vi "InitControls.vi"(8 "error in (no error)":errorcluster, 9 "TestCloneAPI Reference":refnum<vi>, 11 "Controls To Enable":T1) -> (0 "error out":errorcluster)   [LabVIEW 2018, in "SpecAnModule.lvlib"]
doc: "This VI disable controls except those specifically enabled by the user."
uses:
  SpecAnModule.lvlib
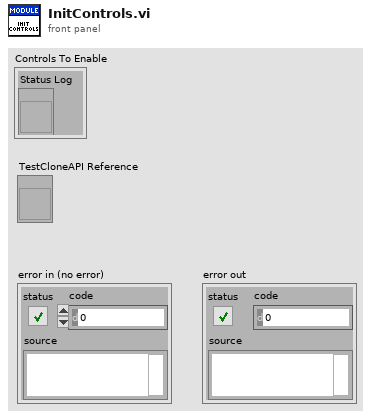
[diagram p1: front panel]
types:
  T1 = cluster{"Status Log":refnum<vi>, "btnAdd":refnum<vi>, "btnStop":refnum<vi>, "Show Panel":refnum<vi>, "btnClear":refnum<vi>}
  T2 = enum8{"Enabled", "Disabled", "Disabled and Grayed Out"}
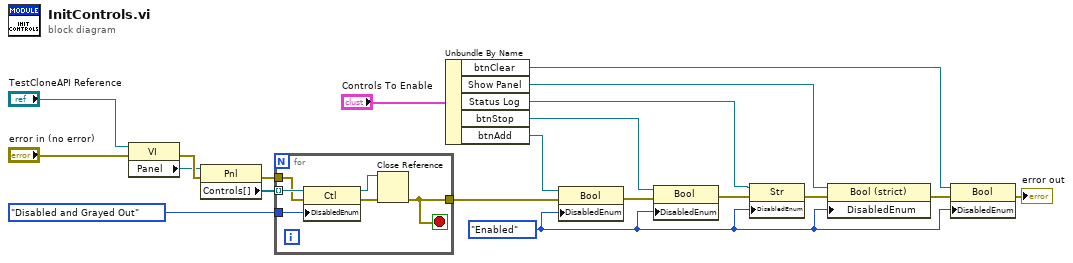
[diagram p0: block diagram]
diagram:
  w7 = T2."Enabled" ("Disabled")
  n1 = property class="VI"(reference="TestCloneAPI Reference", error in="error in (no error)") -> (error out=w17:errorcluster, "Panel"=w14:refnum<vi>)  [unwired: 1 out]
  n2 = property class="Pnl"(reference=w14, error in=w17) -> (error out=w18:errorcluster, "Controls[]"=w15:refnum<vi>[])  [unwired: 1 out]
  n3 = for {
    tunnel: w15 -> [w26] mode=indexing
    tunnel: w18 -> [w25]
    tunnel: [w22] -> w19
    tunnel: T2."Disabled and Grayed Out" ("Disabled") -> [w21]
    stop <- w22 stop-if-true
    n4 = property class="Ctl"(reference=w26, error in=w25, "DisabledEnum"=w21) -> (reference out=w23:refnum<vi>, error out=w24:errorcluster)
    n5 = Close Reference(reference=w23, error in (no error)=w24) -> (error out=w22:errorcluster)
  }
  n6 = Unbundle By Name("Controls To Enable") -> ("btnClear"=w1:refnum<vi>, "Show Panel"=w2:refnum<vi>, "Status Log"=w3:refnum<vi>, "btnStop"=w4:refnum<vi>, "btnAdd"=w5:refnum<vi>)
  n7 = property on="Property Node" class="Bool"(reference=w5, error in=w19, "DisabledEnum"=w7) -> (error out=w12:errorcluster)  [unwired: 1 out]
  n8 = property on="Property Node" class="Bool"(reference=w4, error in=w12, "DisabledEnum"=w7) -> (error out=w11:errorcluster)  [unwired: 1 out]
  n9 = property on="Property Node" class="Str"(reference=w3, error in=w11, "DisabledEnum"=w7) -> (error out=w10:errorcluster)  [unwired: 1 out]
  n10 = property on="Property Node" class="Bool (strict)"(reference=w2, error in=w10, "DisabledEnum"=w7) -> (error out=w9:errorcluster)  [unwired: 1 out]
  n11 = property on="Property Node" class="Bool"(reference=w1, error in=w9, "DisabledEnum"=w7) -> (error out=→"error out":errorcluster)  [unwired: 1 out]
